vi "appendXMLID.vi"(8 "error in (no error)":errorcluster, 9 "ID":i32, 10 "Parent Device Node":refnum<k20>, 11 "DOM document in":refnum<k20>) -> (0 "error out":errorcluster)   [LabVIEW 2013]
uses:
  <resource>/objmgr/DOMUserDefRef.rc
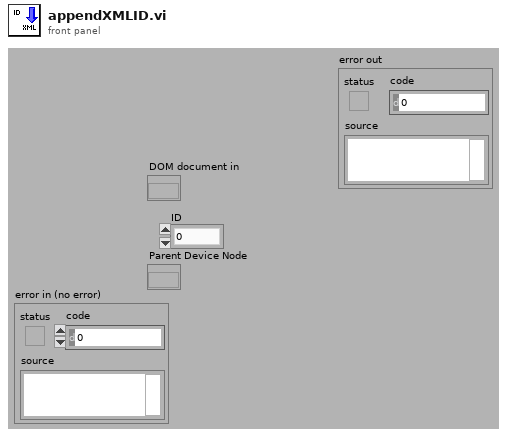
[diagram p1: front panel]
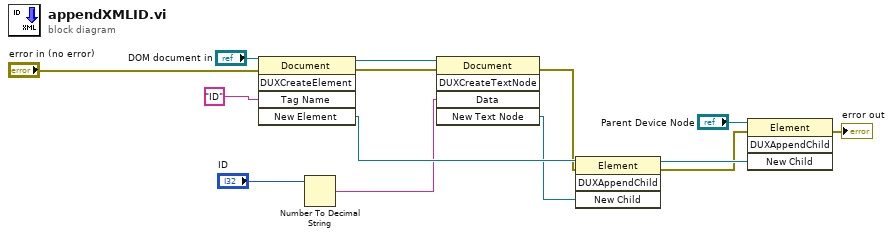
[diagram p0: block diagram]
diagram:
  n1 = invoke class="Document" method="DUXCreateElement"(reference="DOM document in", error in="error in (no error)", "Tag Name"="ID") -> (reference out=w13:refnum<k20>, error out=w6:errorcluster, "New Element"=w11:refnum<k20>)  [unwired: 2 in, 2 out]
  n2 = Number To Decimal String(number="ID") -> (decimal integer string=w1:string)  [unwired: 1 in]
  n3 = invoke class="Document" method="DUXCreateTextNode"(reference=w13, error in=w6, "Data"=w1) -> (error out=w5:errorcluster, "New Text Node"=w10:refnum<k20>)  [unwired: 2 in, 3 out]
  n4 = invoke class="Element" method="DUXAppendChild"(reference=w11, error in=w5, "New Child"=w10) -> (reference out=w8:refnum<k20>, error out=w4:errorcluster)  [unwired: 1 in, 2 out]
  n5 = invoke class="Element" method="DUXAppendChild"(reference="Parent Device Node", error in=w4, "New Child"=w8) -> (error out=→"error out":errorcluster)  [unwired: 1 in, 3 out]
